vi "stable current.vi"() -> ()   [LabVIEW 2016]
uses:
  <resource>/objmgr/daqmx.rc
  <vilib>/DAQmx/read.llb/DAQmx Read (Analog 1D DBL 1Chan NSamp).vi
  <vilib>/DAQmx/write.llb/DAQmx Write (Digital Wfm 1Chan NSamp).vi
  <vilib>/Analysis/NI_AALBase.lvlib
  <vilib>/Analysis/baseanly.llb/Mean (DBL).vi
panel:
  out "error out 4":errorcluster
  in  "error out 2":errorcluster
  in  "stop 2":bool
  out "Numeric":i32
  out "mean":dbl format="%0.8f"
  out "Waveform Chart 2":dbl(graph)
  out "x-y 2":u32
  out "x-y":u32
  out "millisecond timer value":u32
  out "size(s) 2":i32
  out "Histogram":dynamicdata(graph)
  out "Waveform Chart":dbl(graph)
  out "error out":errorcluster
  in  "stop":bool
  out "subarray":dbl[](array[numeric])
  out "error out 3":errorcluster
  out "error out 6":errorcluster
  in  "task/channels in":refnum<k21>="testcurrent"
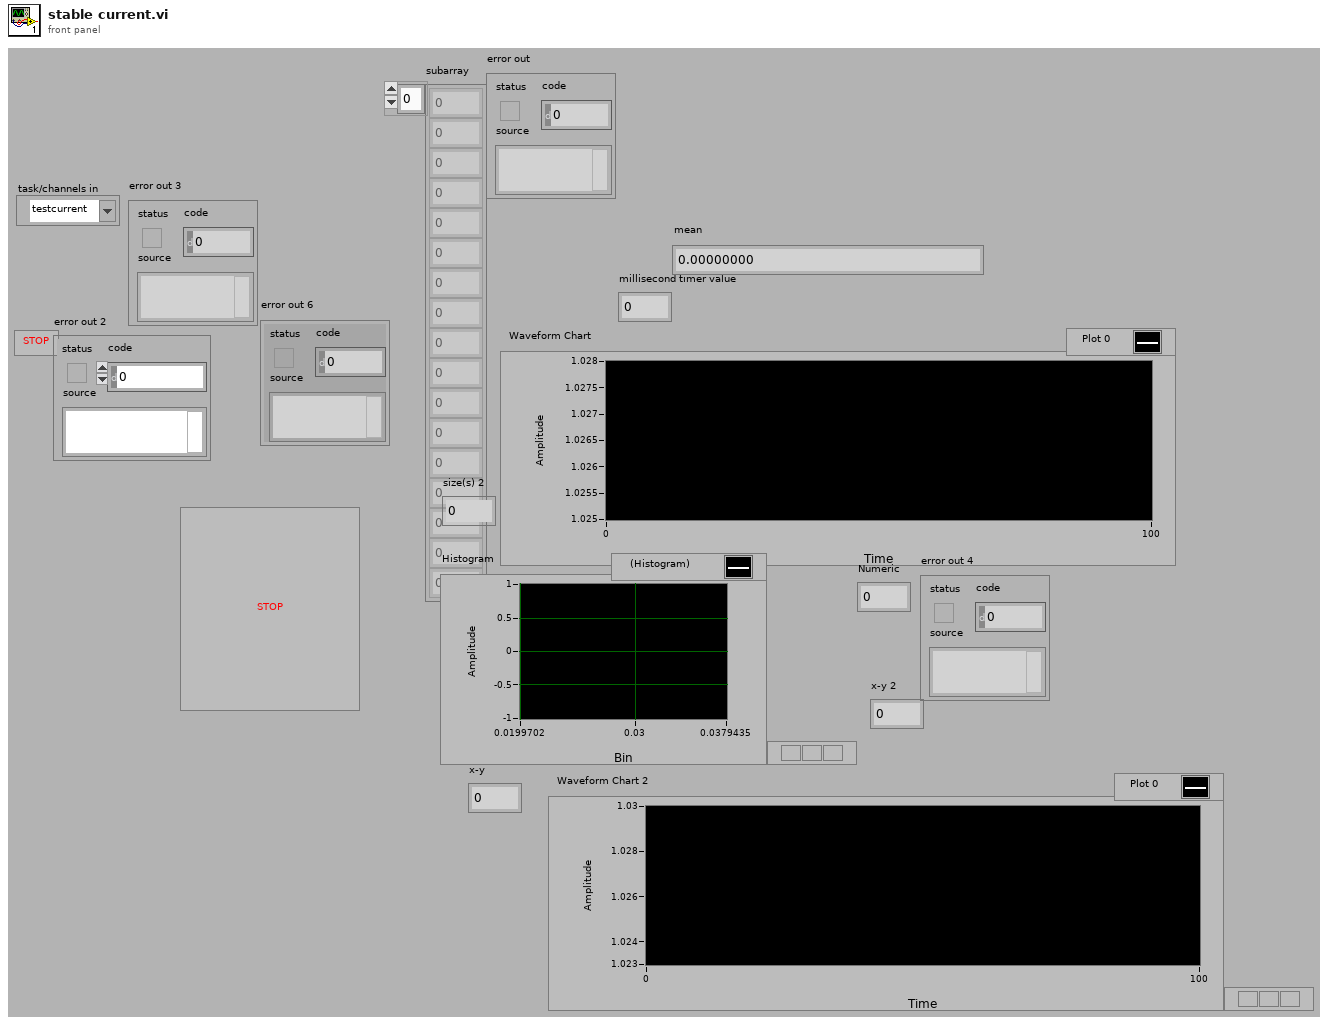
[diagram p1: front panel]
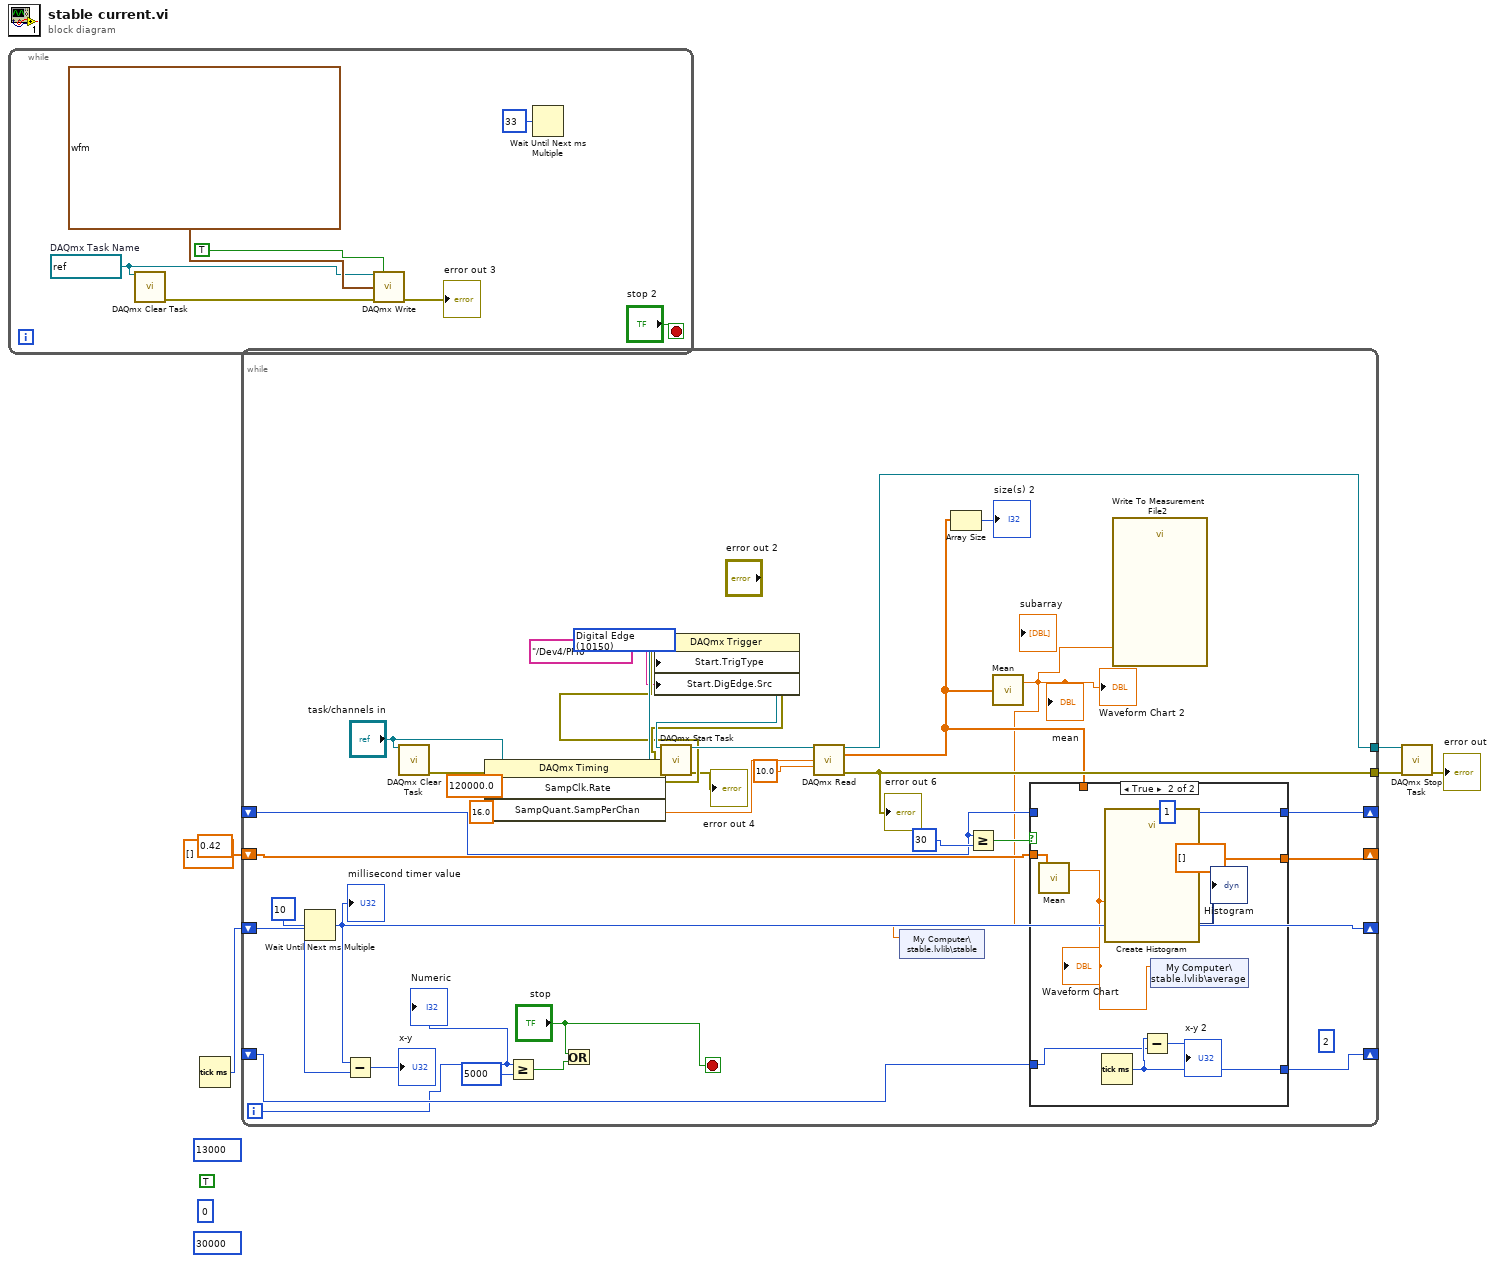
[diagram p0: block diagram]
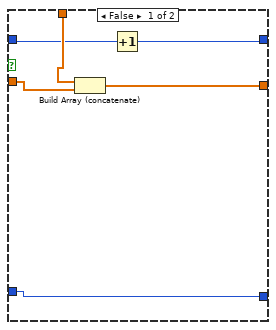
[diagram p2: hidden frame]
diagram:
  (unwired) 0.42 ("mean")
  (unwired) u32 0 ("buffer size (in samples per channel)")
  (unwired) u32 13000 ("buffer size (in samples per channel)")
  (unwired) u32 30000 ("buffer size (in samples per channel)")
  (unwired) TRUE ("auto start")
  n1 = while {
    stop <- "stop 2" stop-if-true
    w11 = refnum<k21> "chop2"  # DAQmx Task Name
    n2 = call <vilib>:"DAQmx Clear Task.vi"("task in"=w11) -> ("error out"=w9:errorcluster)  [unwired: 14 in]
    n3 = call-poly <vilib>:"DAQmx Write.vi"("task/channels in"=w11, "auto start"=TRUE, "data"=digitalwaveform {"t0"=timestamp(0 s since 1904-01-01), "dt"=0.0001, "Y"={"transitions"=[], "data"=array1150x16[18400 elements]}} ("digital waveform"), "error in"=w9) -> ("error out"=→"error out 3":errorcluster)  [unwired: 9 in, 2 out]
    n4 = Wait Until Next ms Multiple(millisecond multiple=u32 33) -> ()  [unwired: 1 out]
  }
  n5 = Tick Count (ms)() -> (millisecond timer value=w3:u32)
  n6 = while {
    tunnel: [w46] -> w5
    tunnel: [w45] -> w2
    shift-right: [w21] -> _
    shift-left: w3 -> [w42]
    shift-right: [w33] -> _
    shift-left: dbl[] [] -> [w32]
    shift-right: [w30] -> _
    shift-left: _ -> [w29]
    shift-right: [w28] -> _
    shift-left: _ -> [w27]
    i -> [w25]
    stop <- "stop" stop-if-true
    w14 = 10150 items=["Analog Edge"=10099, "Digital Edge"=10150, "Digital Pattern"=10398, "Analog Window"=10103, "None"=10230] ("Start.TrigType")
    w35 = 16.0 ("SampClk.Rate")
    (unwired) 2 ("index (row)")
    n7 = Wait Until Next ms Multiple(millisecond multiple=u32 10) -> (millisecond timer value=w21:u32)
    "millisecond timer value" <- w21
    n8 = Subtract(x=w21, y=w42) -> (x-y=→"x-y":u32)
    n9 = call <vilib>:"DAQmx Clear Task.vi"("task in"="task/channels in") -> ("error out"=w40:errorcluster)  [unwired: 14 in]
    n10 = property class="DAQmx Timing"(reference="task/channels in", error in=w40, "SampClk.Rate"=120000.0, "SampQuant.SampPerChan"=w35) -> (reference out=w19:refnum<k21>, error out=w16:errorcluster)
    n11 = Greater Or Equal?(x=w25, y=5000) -> (x >= y?=w24:bool)
    n12 = Or(x="stop", y=w24) -> ()  [unwired: 1 out]
    n13 = property class="DAQmx Trigger"(reference=w19, error in=w16, "Start.TrigType"=w14, "Start.DigEdge.Src"=tag "/Dev4/PFI0") -> (reference out=w18:refnum<k21>, error out=w17:errorcluster)
    n14 = call <vilib>:"DAQmx Start Task.vi"("task/channels in"=w18, "error in"=w17) -> ("task out"=w37:refnum<k21>, "error out"=→"error out 4":errorcluster)  [unwired: 12 in]
    n15 = call-poly <vilib>:"DAQmx Read.vi"("task/channels in"=w37, "number of samples per channel"=w35, "timeout"=10.0) -> ("task out"=w45:refnum<k21>, "data"=w26:dbl[], "error out"=w46:errorcluster)  [unwired: 10 in]
    "error out 6" <- w46
    n16 = Array Size(array=w26) -> (size(s)=→"size(s) 2":i32)
    n17 = Greater Or Equal?(x=w29, y=30 ("index (row)")) -> (x >= y?=w34:bool)
    n18 = call-poly <vilib>:"Mean.vi"("X"=w26) -> ("mean"=w20:dbl)  [unwired: 1 out]
    "Waveform Chart 2" <- w20
    "mean" <- w20
    n19 = shared-variable "My Computer\\stable.lvlib\\stable"(w20) -> ()  [unwired: 1 in, 1 out]
    n20 = case shown="True" w34 {
      tunnel: w26 -> [w52 _]
      tunnel: [w51 dbl[] []] -> w33
      tunnel: w32 -> [w50 w57]
      tunnel: [w48 1 ("index (row)")] -> w30
      tunnel: w29 -> [w49 _]
      tunnel: [w47 w56] -> w28
      tunnel: w27 -> [w47 w55]
      frame False {
        n21 = Build Array (concatenate)(w52, w50) -> (w51:dbl[])
        n22 = Increment(x=w49) -> (x+1=w48:i32)
      }
      frame True {
        n23 = call-poly <vilib>:"Mean.vi"("X"=w57) -> ("mean"=w53:dbl)  [unwired: 1 out]
        "Waveform Chart" <- w53
        n24 = Tick Count (ms)() -> (millisecond timer value=w56:u32)
        n25 = call "Create Histogram"("Signal"=w53) -> ("Histogram"=→"Histogram":dynamicdata)  [unwired: 9 in, 1 out]
        n26 = Subtract(x=w56, y=w55) -> (x-y=→"x-y 2":u32)
        n27 = shared-variable "My Computer\\stable.lvlib\\average"(w53) -> ()  [unwired: 1 in, 1 out]
      }
    }
    n28 = call "Write To Measurement File2"("Signals"=w20) -> ()  [unwired: 16 in, 3 out]
    "Numeric" <- w25
  }
  n29 = call <vilib>:"DAQmx Stop Task.vi"("task/channels in"=w2, "error in"=w5) -> ("error out"=→"error out":errorcluster)  [unwired: 12 in, 1 out]
